vi "Heise Barometric Pressure 901A Raw String.vi"(11 "Data Stream":string) -> (2 "Units":string, 3 "Barometric Pressure":string)   [LabVIEW 2023]
uses:
  <vilib>/Utility/error.llb/whitespace.ctl
  <vilib>/Utility/error.llb/Trim Whitespace One-Sided.vi
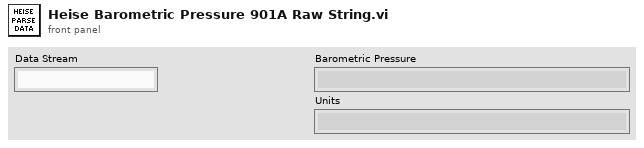
[diagram p1: front panel]
types:
  T1 = typedef "whitespace.ctl" = u16
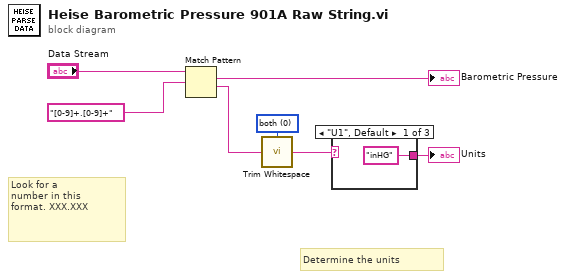
[diagram p0: block diagram]
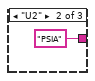
[diagram p2: hidden frame]
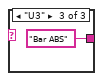
[diagram p3: hidden frame]
diagram:
  w4 = T1 0 items=["both", "start of string", "end of string"] ("location (both)")
  # "Determine the units"
  # "Look for a \nnumber in this \nformat. XXX.XXX"
  n1 = Match Pattern(string="Data Stream", regular expression="[0-9]+.[0-9]+") -> (match substring=→"Barometric Pressure":string, after substring=w5:string)  [unwired: 1 in, 2 out]
  n2 = call <vilib>:"Trim Whitespace.vi"("string"=w5, "location (both)"=w4) -> ("trimmed string"=w3:string)
  n3 = case shown="\"U1\", Default" w3 {
    tunnel: ["inHG" "PSIA" "Bar ABS"] -> w2
    frame "U1", Default {
    }
    frame "U2" {
    }
    frame "U3" {
    }
  }
  "Units" <- w2
